vi "Melody Player EQ Analyzed.vi"(9 "Sound Device":u32(ring) items=["Default (0)", "Device 1", "Device 2", "Device 3", "Device 4"], 10 "Play":bool, 11 "Melody Type":T1(ring)) -> (0 "error out":errorcluster, 2 "EQ Magnitude Graph":cluster{"X":dbl, "Y":dbl}[](graph), 3 "Raw Waveform Graph":dbl[](graph))   [LabVIEW 2026]
doc: "Native LabVIEW melody player with low-level sound output and frequency-component based EQ graph."
uses:
  <vilib>/addons/_NISVFA/_Baseband FFT/SVPO Power Spectrum (1 Ch DBL Array).vi
  <vilib>/addons/_NISVFA/_Baseband FFT/subVIs/svfa_Convert to One-Sided Power Spectrum.vi
  <vilib>/Analysis/2dsp.llb/Power Spectrum.vi
  <vilib>/Analysis/2dsp.llb/Power Spectrum (DBL).vi
  <vilib>/addons/_NISVFA/_Shared subVIs/Windowing/svfa_Scaled Time Domain Window (Array).vi
  <vilib>/addons/_NISVFA/_Spectrum Processing/subVIs/svfa_Spectrum Info Window to windowTd Type Def.vi
  <vilib>/Analysis/4window.llb/Force Window.vi
  <vilib>/Analysis/4window.llb/Force Window (DBL).vi
  <vilib>/Analysis/4window.llb/Exponential Window.vi
  <vilib>/Analysis/4window.llb/Exponential Window (DBL).vi
  <vilib>/Analysis/0measdsp.llb/Scaled Time Domain Window.vi
  <vilib>/Analysis/0measdsp.llb/Scaled Time Domain Window (DBL).vi
  <vilib>/Utility/error.llb/Error Cluster From Error Code.vi
  <vilib>/sound2/lvsound2.llb/Sound Output Write (DBL Single).vi
panel:
  in  "stop":bool
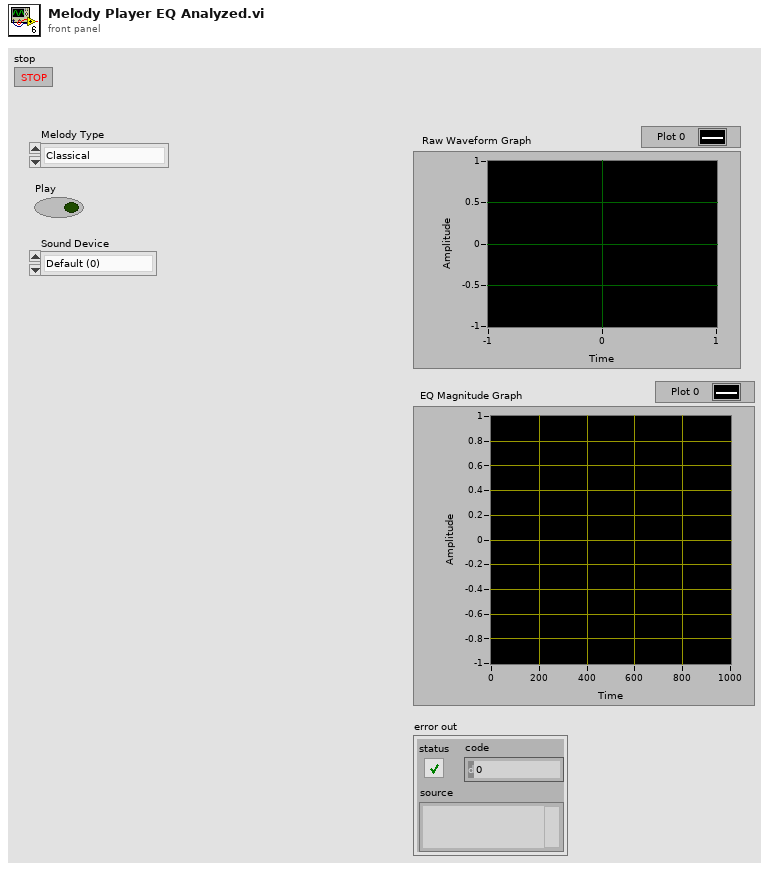
[diagram p1: front panel]
types:
  T1 = enum16{"Classical", "Jazz", "Blues", "Electronic", "Folk"}
  T2 = cluster{"waveform":dbl[], "sample rate (S/s)":dbl}
  T3 = cluster{"sample rate (S/s)":dbl, "number of channels":i32, "bits per sample":i32}
  T4 = typedef "Sound Output Task ID.ctl" = u32
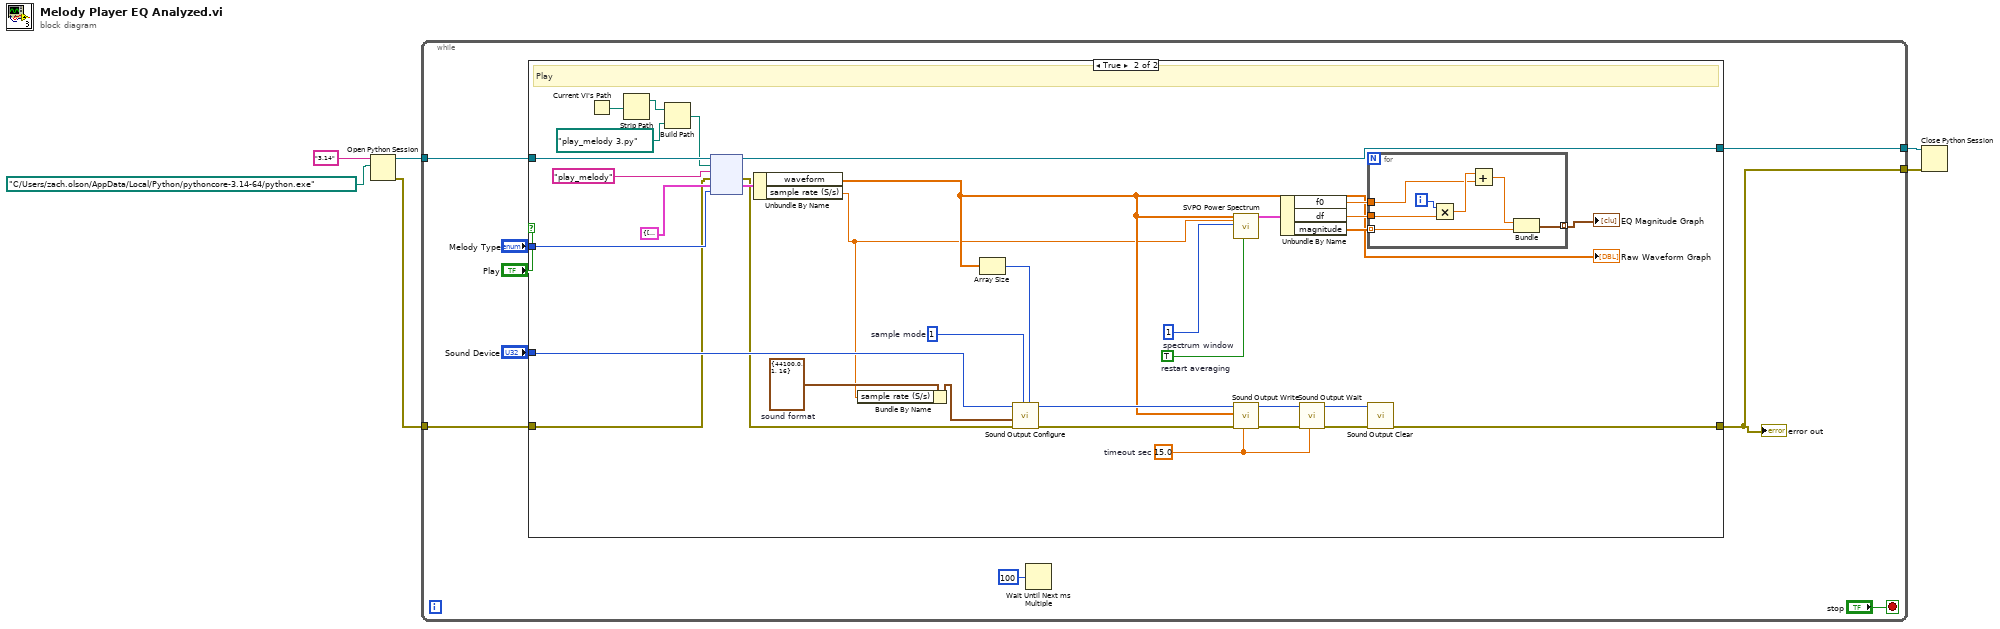
[diagram p0: block diagram]
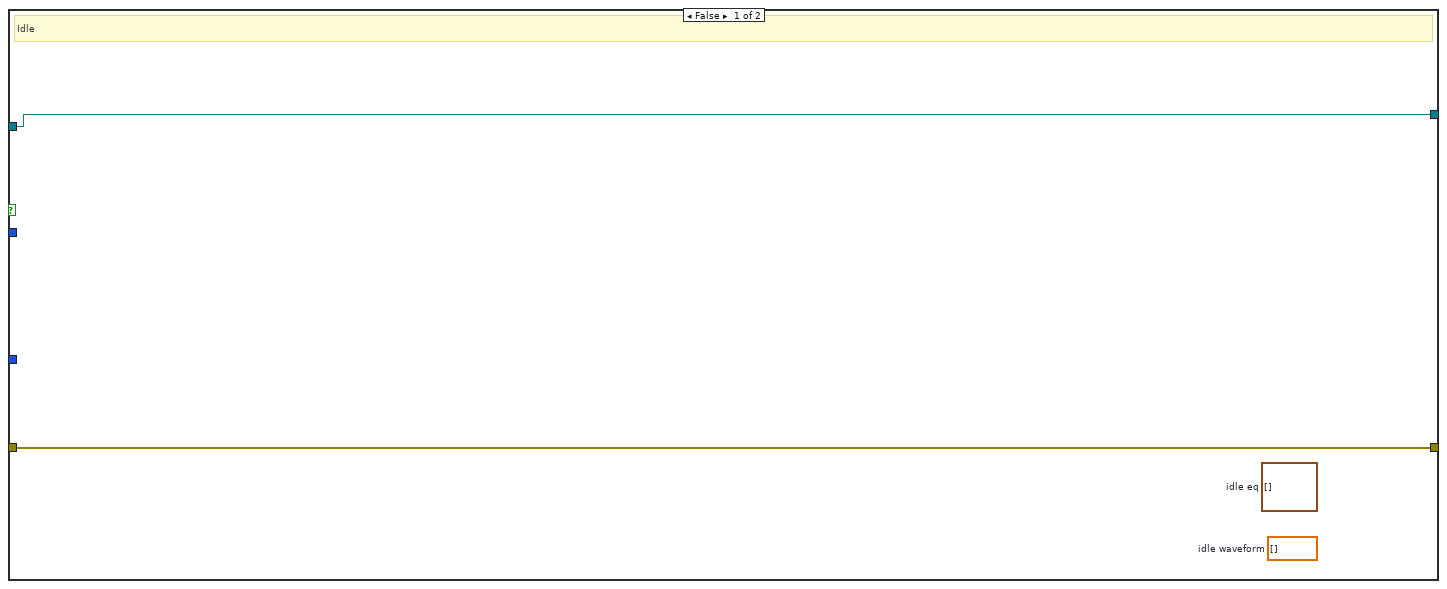
[diagram p2: hidden frame]
diagram:
  n1 = Open Python Session(python version="3.14" ("Python version"), python path=path "C:/Users/zach.olson/AppData/Local/Python/pythoncore-3.14-64/python.exe" ("Python path")) -> (session out=w4:refnum<k35>, error out=w1:errorcluster)  [unwired: 1 in]
  n2 = while {
    tunnel: w4 -> [w12]
    tunnel: [w11] -> w3
    tunnel: [w10] -> w2
    tunnel: w1 -> [w7]
    stop <- "stop" stop-if-true
    n3 = case shown="True" "Play" {
      tunnel: "Melody Type" -> [_ w30]
      tunnel: "Sound Device" -> [_ w45]
      tunnel: w7 -> [w17 w23]
      tunnel: [w17 w35] -> w10
      tunnel: w12 -> [w16 w33]
      tunnel: [w16 w24] -> w11
      frame False {
        (unwired) cluster{"X":dbl, "Y":dbl}[] []  # idle eq
        (unwired) dbl[] []  # idle waveform
        # "Idle"
      }
      frame True {
        w50 = TRUE  # restart averaging
        w51 = u32 1  # spectrum window
        w38 = 15.0  # timeout sec
        w43 = 1  # sample mode
        w44 = T3 {"sample rate (S/s)"=44100.0, "number of channels"=1, "bits per sample"=16}  # sound format
        # "Play"
        n4 = Current VI's Path() -> (path=w19:path)
        n5 = Strip Path(path=w19) -> (stripped path=w18:path)  [unwired: 1 out]
        n6 = Build Path(base path=w18, name or relative path=path "play_melody 3.py" ("module path")) -> (appended path=w20:path)
        n7 = node(w33, w20, "play_melody" ("function name"), w23, T2 {"waveform"=[0.0], "sample rate (S/s)"=22050.0}, w30) -> (w24:refnum<k35>, w22:errorcluster, w29:T2)  [unwired: 1 in, 2 out]
        n8 = Unbundle By Name(w29) -> ("waveform"=w28:dbl[], "sample rate (S/s)"=w25:dbl)
        "Raw Waveform Graph" <- w28
        n9 = Bundle By Name(cluster=w44, "sample rate (S/s)"=w25) -> (w26:T3)
        n10 = Array Size(array=w28) -> (size(s)=w27:i32)
        n11 = call <vilib>:"Sound Output Configure.vi"("number of samples/ch"=w27, "sample mode"=w43, "error in (no error)"=w22, "sound format"=w26, "device ID"=w45) -> ("error out"=w41:errorcluster, "task ID"=w42:T4)  [unwired: 5 in]
        n12 = call-poly <vilib>:"SVPO Power Spectrum.vi"("scaled signal [EU]"=w28, "sampling rate [Hz]"=w25, "window"=w51, "restart averaging? (F)"=w50) -> ("power spectrum [EU^2 rms]"=w49:cluster{"f0":dbl, "df":dbl, "magnitude":dbl[]})  [unwired: 13 in, 2 out]
        n13 = call-poly <vilib>:"Sound Output Write.vi"("timeout (sec)"=w38, "error in (no error)"=w41, "data"=w28, "task ID"=w42) -> ("error out"=w39:errorcluster, "task ID out"=w40:T4)  [unwired: 6 in]
        n14 = Unbundle By Name(w49) -> ("f0"=w47:dbl, "df"=w46:dbl, "magnitude"=w48:dbl[])
        n15 = call <vilib>:"Sound Output Wait.vi"("timeout (sec)"=w38, "error in (no error)"=w39, "task ID"=w40) -> ("error out"=w36:errorcluster, "task ID out"=w37:T4)  [unwired: 7 in]
        n16 = for {
          tunnel: w48 -> [w54] mode=indexing
          tunnel: w47 -> [w56]
          tunnel: w46 -> [w58]
          tunnel: [w53] -> w34 mode=indexing
          i -> [w52]
          n17 = Multiply(x=w52, y=w58) -> (x*y=w57:dbl)
          n18 = Add(x=w57, y=w56) -> (x+y=w55:dbl)
          n19 = Bundle(w55, w54) -> (w53:cluster{dbl, dbl})  [unwired: 1 in]
        }
        "EQ Magnitude Graph" <- w34
        n20 = call <vilib>:"Sound Output Clear.vi"("error in (no error)"=w36, "task ID"=w37) -> ("error out"=w35:errorcluster)  [unwired: 9 in]
      }
    }
    "error out" <- w10
    n21 = Wait Until Next ms Multiple(millisecond multiple=u32 100) -> ()  [unwired: 1 out]
  }
  n22 = Close Python Session(session in=w3, error in=w2) -> ()  [unwired: 1 out]
